vi "GDSAPI_Example_CloneMethods.vi"() -> ()   [LabVIEW 2014]
uses:
  <resource>/Framework/Providers/Open_GDS/API/GDSAPI_CreateClassType.ctl
  <resource>/Framework/Providers/Open_GDS/API/GDSAPI_SubVIs/GDSAPI_ClassProviderType.ctl
  <resource>/Framework/Providers/Open_GDS/API/GDSAPI_SubVIs/GDSAPI_ClassTemplateType.ctl
  <resource>/Framework/Providers/Open_GDS/ClassProviders/Common/String/GDSString_MethodDescriptionType.ctl
  <resource>/Framework/Providers/Open_GDS/ClassProviders/Common/CommonVIs/CommonVIs_AttributeType.ctl
  <resource>/Framework/Providers/Open_GDS/ClassProviders/Common/CommonVIs/CommonVIs_AttributeDataType.ctl
  <resource>/Framework/Providers/Open_GDS/ClassProviders/Common/String/GDSString_AccessScopeModifierType.ctl
  <resource>/Framework/Providers/Open_GDS/ClassProviders/Common/String/GDSString_ModifierType.ctl
  <resource>/Framework/Providers/Open_GDS/ClassProviders/Common/CommonVIs/CommonVIs_PropertyType.ctl
  <resource>/Framework/Providers/Open_GDS/ClassProviders/Provider_EndevoGOOP300/GOOP300_SubVIs/GOOP300_MethodScopeType.ctl
  <resource>/Framework/Providers/Open_GDS/API/GDSAPI_SubVIs/GDSAPI_MethodType.ctl
panel:
  in  "Clone(T)/CreateBasedOnOverrideMethod(F)":bool
  out "error out":errorcluster
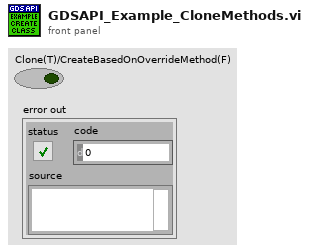
[diagram p1: front panel]
types:
  T1 = typedef "GOOP300_MethodScopeType.ctl" = enum16{"Use Parent Folder Scope", "Public", "Protected", "Private", "Community"}
  T2 = typedef "GDSAPI_MethodType.ctl" = enum16{"Read Attribute", "Write Attribute", "Read & Write Attribute", "None Modifying Method", "Get Property", "Set Property", "Read Property", "Write Property", "Static Method", "Interface Method"}
  T3 = cluster{"MethodName":string, "RelativeMethodPath":path, "MethodDescription":string, "Scope/Visibility":T1, "MethodType":T2, "RelativeProjectClassPath":string, "DynamicDispatchVi":bool, "OverrideMethod(Path)/PropertyMethod(AttributeName)":string}
  T4 = typedef "GDSString_MethodDescriptionType.ctl" = cluster{"ReturnType":T5, "MethodName":string, "AccessScope":T7, "Modifiers":T8[], "MethodDocumentation":string, "MethodContent":string, "MethodArguments":T5[], "GetProperty":T9, "SetProperty":T9}
  T5 = typedef "CommonVIs_AttributeType.ctl" = cluster{"Name":string, "DataType":T6, "ArrayDim":i32, "CtrlPath":path, "DataTypeString":string, "AccessScope":T7, "InitialData":variant}
  T6 = typedef "CommonVIs_AttributeDataType.ctl" = enum16{"UINT8", "INT8", "UINT16", "INT16", "UINT32", "INT32", "UINT64", "INT64", "SGL", "DBL", "EXT", "CSG", "CDB", "CXT", "TimeStamp", "STRING", "PATH", "BOOL", "ENUM", "RefNum", "VIRefNum", "LabVIEW Class", "Cluster", "Variant", "TypeDef", "Waveform", "LabVIEW Object", "Other", "void"}
  T7 = typedef "GDSString_AccessScopeModifierType.ctl" = enum16{"public", "private", "protected", "internal"}
  T8 = typedef "GDSString_ModifierType.ctl" = enum16{"abstract", "static", "final", "synchronized", "strictfp", "async", "const", "event", "extern", "new", "native ", "override", "partial", "readonly", "sealed", "unsafe", "virtual", "volatile"}
  T9 = typedef "CommonVIs_PropertyType.ctl" = cluster{"Active":bool, "AccessScope":T7, "Code":string}
  T10 = typedef "GDSAPI_CreateClassType.ctl" = cluster{"ClassProvider":T11, "NewClassFolder":path, "ParentLvClassFilePath":path, "ClassName":string, "ClassDescription":string, "ClassTemplate":T12}
  T11 = typedef "GDSAPI_ClassProviderType.ctl" = enum16{"LabVIEW Native(By value)", "GOOP-3(By reference)", "GOOP-4(By reference)"}
  T12 = typedef "GDSAPI_ClassTemplateType.ctl" = enum16{"Standard", "Singleton", "Interface(By Aggregation)", "Interface(By VI Server)"}
  T13 = cluster{"MethodName":string, "RelativeMethodPath":path, "MethodDescription":string, "Scope/Visibility":T1, "MethodType":T2, "RelativeProjectClassPath":string, "DynamicDispatchVi":bool, "OverrideMethod(Path)/PropertyMethod(AttributeName)":string}[]
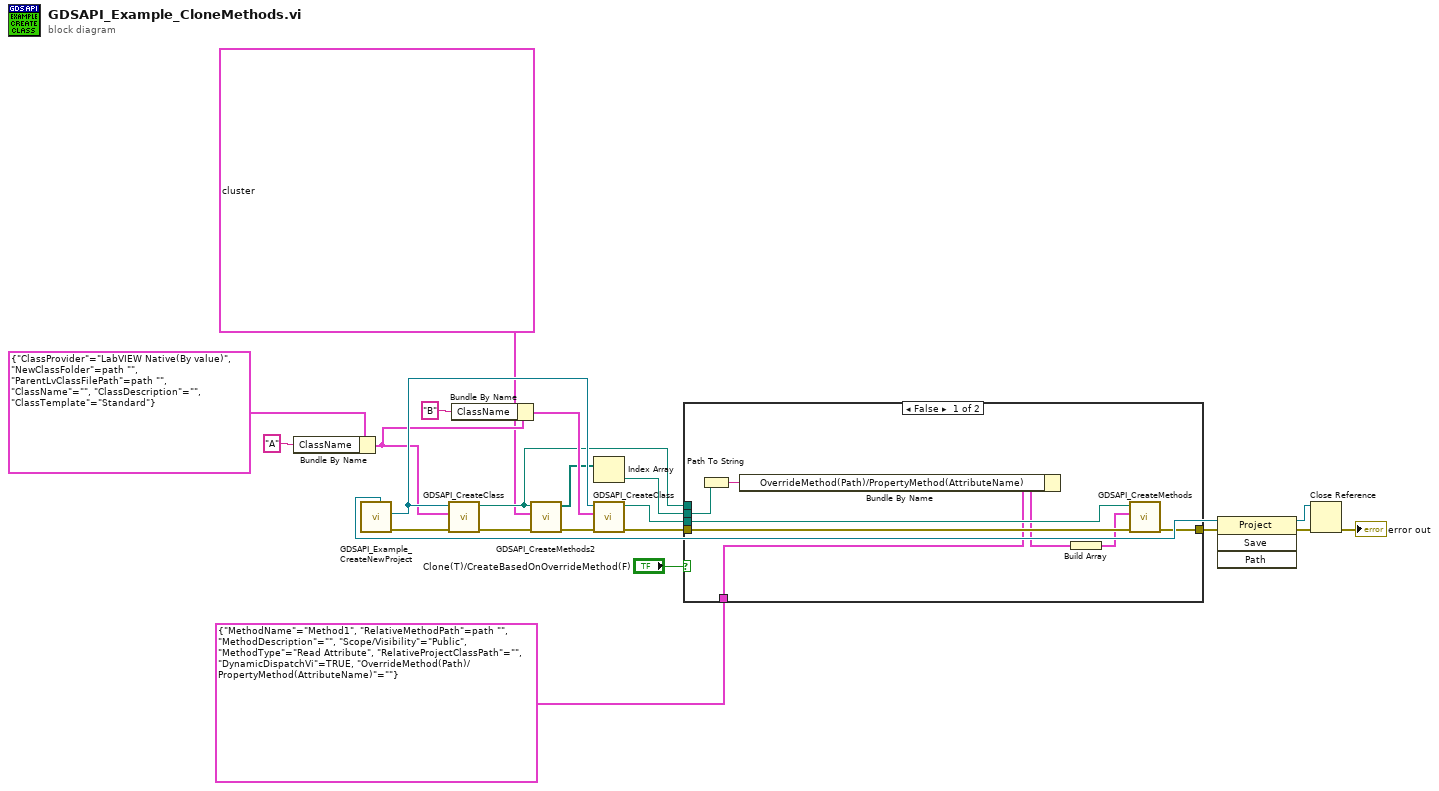
[diagram p0: block diagram]
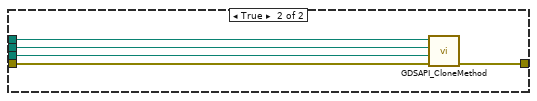
[diagram p2: hidden frame]
diagram:
  n1 = Bundle By Name(cluster=T10 {"ClassProvider"=enum."LabVIEW Native(By value)", "NewClassFolder"=path "", "ParentLvClassFilePath"=path "", "ClassName"="", "ClassDescription"="", "ClassTemplate"=enum."Standard"} ("CreateClassType"), "ClassName"="A") -> (w14:T10)
  n2 = call <resource>:"GDSAPI_Example_CreateNewProject.vi"() -> ("error out"=w22:errorcluster, "ProjectItem out"=w21:refnum<vi>, "ProjectRefOut"=w17:refnum<vi>)  [unwired: 8 in, 1 out]
  n3 = call <resource>:"GDSAPI_CreateClass.vi"("error in (no error)"=w22, "CreateClassType"=w14, "ProjectItem"=w21) -> ("error out"=w12:errorcluster, "LvClassFileOut"=w7:path)  [unwired: 6 in, 1 out]
  n4 = Bundle By Name(cluster=w14, "ClassName"="B") -> (w15:T10)
  n5 = call <resource>:"GDSAPI_CreateMethods2.vi"("error in (no error)"=w12, "Methods"=T4[] [{"ReturnType"={"Name"="Out 1", "DataType"=enum."UINT8", "ArrayDim"=0, "CtrlPath"=path "", "DataTypeString"="", "AccessScope"=enum."public", "InitialData"=variant}, "MethodName"="Method1", "AccessScope"=enum."public", "Modifiers"=[], "MethodDocumentation"="", "MethodContent"="", "MethodArguments"=[{"Name"="In 1", "DataType"=enum."UINT8", "ArrayDim"=0, "CtrlPath"=path "", "DataTypeString"="", "AccessScope"=enum."public", "InitialData"=variant}, {"Name"="In 2", "DataType"=enum."STRING", "ArrayDim"=0, "CtrlPath"=path "", "DataTypeString"="", "AccessScope"=enum."public", "InitialData"=variant}], "GetProperty"={"Active"=FALSE, "AccessScope"=enum."public", "Code"=""}, "SetProperty"={"Active"=FALSE, "AccessScope"=enum."public", "Code"=""}}], "ClassPath(*.lvclass)"=w7) -> ("error out"=w13:errorcluster, "MethodsCreated"=w4:path[])  [unwired: 7 in]
  n6 = Index Array(array=w4) -> (element=w3:path)  [unwired: 1 in]
  n7 = call <resource>:"GDSAPI_CreateClass.vi"("error in (no error)"=w13, "CreateClassType"=w15, "ProjectItem"=w21) -> ("error out"=w9:errorcluster, "LvClassFileOut"=w6:path)  [unwired: 6 in, 1 out]
  n8 = case shown="False" "Clone(T)/CreateBasedOnOverrideMethod(F)" {
    tunnel: w9 -> [w30 w35]
    tunnel: [w29 w34] -> w8
    tunnel: w7 -> [_ w33]
    tunnel: w6 -> [w28 w32]
    tunnel: w3 -> [w23 w31]
    tunnel: T3 {"MethodName"="Method1", "RelativeMethodPath"=path "", "MethodDescription"="", "Scope/Visibility"=enum."Public", "MethodType"=enum."Read Attribute", "RelativeProjectClassPath"="", "DynamicDispatchVi"=TRUE, "OverrideMethod(Path)/PropertyMethod(AttributeName)"=""} ("CreateMethodData") -> [w26 _]
    frame False {
      n9 = Path To String(path=w23) -> (string=w24:string)
      n10 = Bundle By Name(cluster=w26, "OverrideMethod(Path)/PropertyMethod(AttributeName)"=w24) -> (w25:T3)
      n11 = Build Array(w25) -> (w27:T13)
      n12 = call <resource>:"GDSAPI_CreateMethods.vi"("error in (no error)"=w30, "Methods"=w27, "ClassPath(*.lvclass)"=w28) -> ("error out"=w29:errorcluster)  [unwired: 7 in, 1 out]
    }
    frame True {
      n13 = call <resource>:"GDSAPI_CloneMethod.vi"("error in (no error)"=w35, "DestinationClassPath(*.lvclass)"=w32, "SourceClassMethod(*.vi)"=w31, "SourceClassPath(*.lvclass)"=w33) -> ("error out"=w34:errorcluster)  [unwired: 6 in, 1 out]
    }
  }
  n14 = invoke class="Project" method="Save"(reference=w17, error in=w8) -> (reference out=w19:refnum<vi>, error out=w20:errorcluster)  [unwired: 2 in, 2 out]
  n15 = Close Reference(reference=w19, error in (no error)=w20) -> (error out=→"error out":errorcluster)
